vi "vesselMonitor.vi"() -> ()   [LabVIEW 2014]
panel:
  out "e_i":cluster{"Numeric":dbl, "Numeric":dbl}(graph)
  out "e_b":cluster{"Numeric":dbl, "Numeric":dbl}(graph)
  out "e_psi":dbl(graph)
  in  "stop 2":bool
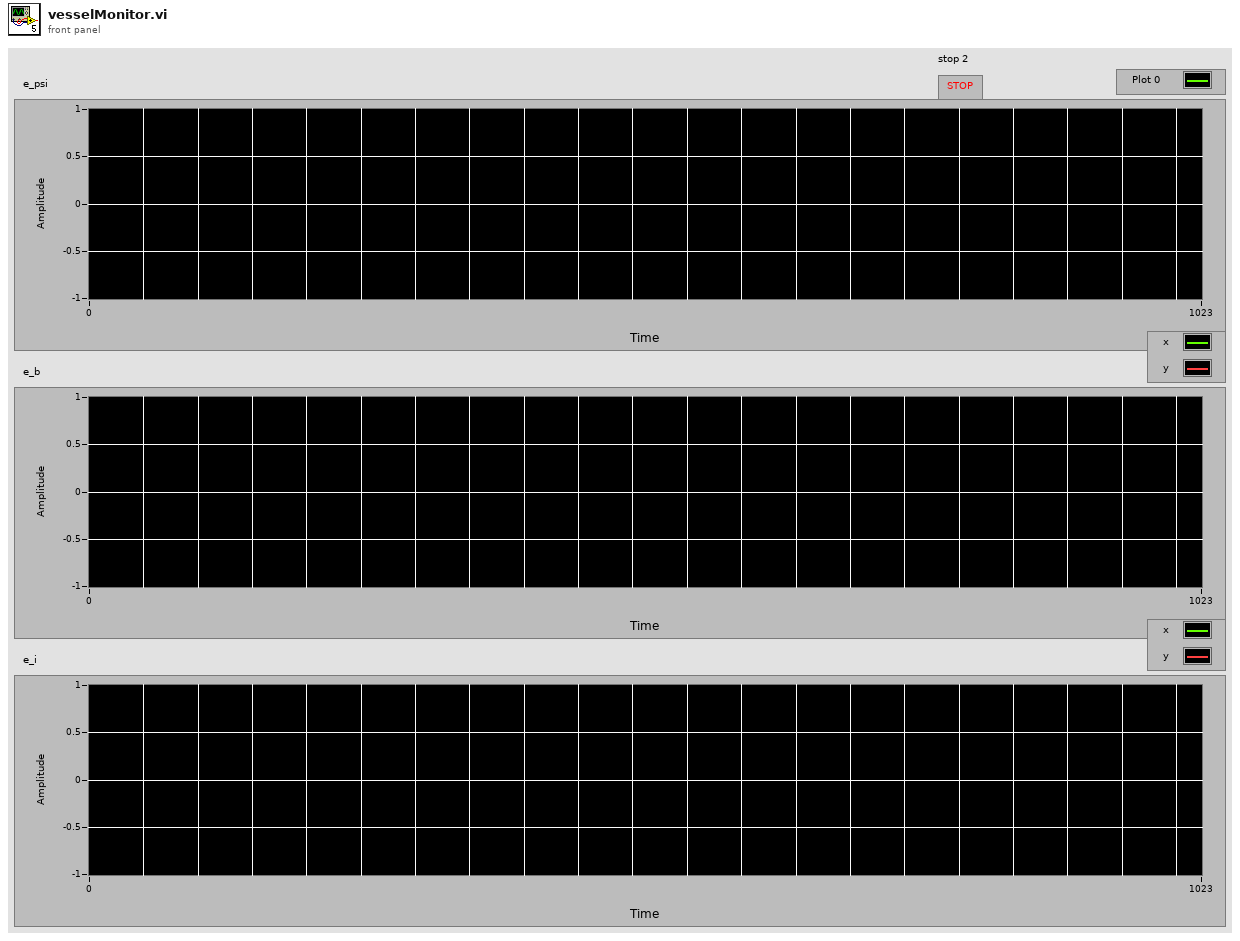
[diagram p1: front panel]
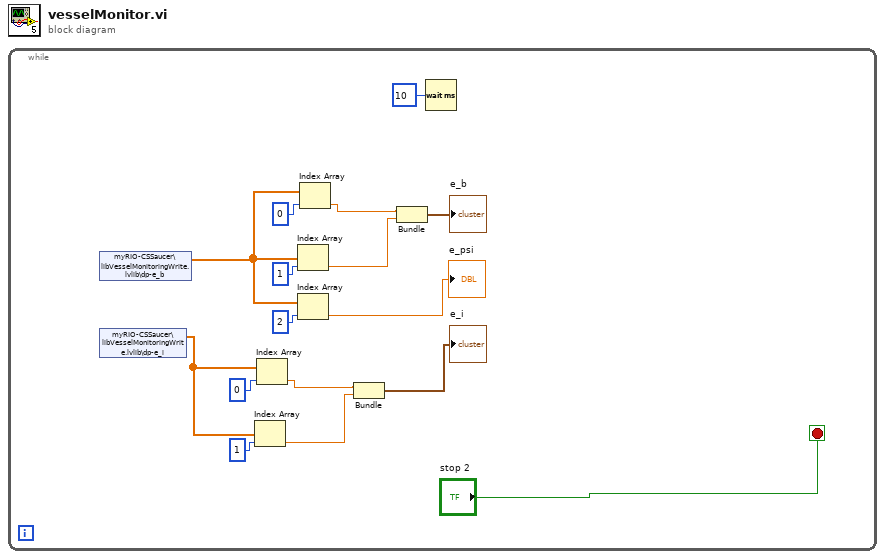
[diagram p0: block diagram]
diagram:
  n1 = while {
    stop <- "stop 2" stop-if-true
    n2 = shared-variable "myRIO-CSSaucer\\libVesselMonitoringWrite.lvlib\\dp-e_b"() -> (w11:dbl[])  [unwired: 1 in, 1 out]
    n3 = shared-variable "myRIO-CSSaucer\\libVesselMonitoringWrite.lvlib\\dp-e_i"() -> (w2:dbl[])  [unwired: 1 in, 1 out]
    n4 = Index Array(array=w2, index=1) -> (element=w3:dbl)
    n5 = Index Array(array=w2, index=0) -> (element=w4:dbl)
    n6 = Index Array(array=w11, index=1) -> (element=w8:dbl)
    n7 = Index Array(array=w11, index=2) -> (element=→"e_psi":dbl)
    n8 = Index Array(array=w11, index=0) -> (element=w9:dbl)
    n9 = Bundle("Numeric"=w4, "Numeric"=w3) -> (→"e_i":cluster{"Numeric":dbl, "Numeric":dbl})  [unwired: 1 in]
    n10 = Bundle("Numeric"=w9, "Numeric"=w8) -> (→"e_b":cluster{"Numeric":dbl, "Numeric":dbl})  [unwired: 1 in]
    n11 = Wait (ms)(milliseconds to wait=u32 10) -> ()  [unwired: 1 out]
  }
